vi "FPGA Top - Packet TX Only.vi"() -> ()   [LabVIEW 2020, in "My Network FPGA v1.lvlib"]
uses:
  My Network FPGA v1.lvlib
  <instrlib>/_niInstr/Network/Types/v1/MAC Address.ctl
  <instrlib>/_niInstr/Network/Types/v1/IPv4 Address.ctl
  <instrlib>/_niInstr/CLIP Adapters/v1/FPGA/AXI4-Lite/FXP32 Address - FXP32 Data/Public/CLIP Resources.ctl
  <vilib>/Platform/TimedLoop/XDataNode/timing_clust.ctl
  <vilib>/Platform/TimedLoop/XDataNode/nitl_modes.ctl
  <vilib>/Platform/TimedLoop/XDataNode/wakeup.ctl
  <instrlib>/_niInstr/Network/Ethernet/MAC/CLIP/v1/1GbE/Resources.ctl
  <instrlib>/_niInstr/FIFO Register Bus/v1/FPGA/niInstr FIFO Register Bus v1 FPGA.lvclass
  p:/lvdist/win32/export/20.0/20.0.0f2/dist/instr.lib/_niInstr/Instruction Framework/v1/FPGA/Interfaces/Instruction Producer/Instruction Producer.lvclass
  <instrlib>/_niInstr/CLIP Adapters/v1/FPGA/AXI4-Lite/Address Space Collection/niInstr AXI4-Lite Address Space Collection v1 FPGA.lvclass
  p:/lvdist/win32/export/20.0/20.0.0f2/dist/instr.lib/_niInstr/Instruction Framework/v1/FPGA/Interfaces/Address Space Collection/Address Space Collection.lvclass
  <vilib>/rvi/Emulation/niFpgaGetClockAttributes.vi
  <vilib>/rvi/Emulation/niFpgaSctlEmulationGetInTimedLoop.vi
  <vilib>/rvi/Emulation/niFpgaEmulationReportErrorSimple.vi
  <vilib>/rvi/Emulation/niFpgaCriticalErrorInLSC.vi
  <vilib>/rvi/DataTransferAndStorage/Container/Common/niFpgaContainerGetUniqueNameForEmu.vi
  <vilib>/rvi/DataTransferAndStorage/Container/Common/niFpgaContainerSetEmuInfo.vi
  <vilib>/rvi/eio/common/nirviEmuReportErrorAndStop.vi
  <vilib>/rvi/Emulation/niFpgaProcessEmulError.vi
  <vilib>/rvi/DataTransferAndStorage/Container/Common/niFpgaContainerExecOnDevCompGetState.vi
  <vilib>/rvi/Emulation/niFpgaEmulationIsFPGAContextNoSignature.vi
  <vilib>/rvi/errors/niFpgaSetErrorForExecOnDevCompSimple.vi
  <vilib>/rvi/FIFO/Fifo_Resource/nirvififoEmulationSetSize.vi
  <vilib>/rvi/FIFO/Fifo_Resource/nirviFifoEmulationQueueMgr.vi
  <instcachedir>/0/nirviFifoEmulationQueueMgr_E5CAEC123FF24DC58D834DCA3CDAA9B5.lvgen/nirviFifoEmulationQueueMgr_E5CAEC123FF24DC58D834DCA3CDAA9B5_022.vi
  <vilib>/rvi/FIFO/Fifo_Resource/nirvififoEmulationDetermineInputValidOut.vi
  <vilib>/rvi/FIFO/Fifo_Resource/nirvififoEmulationCreateLock.vi
  <vilib>/rvi/FIFO/Fifo_Resource/nirvififoEmulationObtainLock.vi
  <vilib>/rvi/FIFO/Fifo_Resource/nirvififoEmulationReleaseLock.vi
  <vilib>/rvi/occurrence/nirviWaitOnOccurrenceBase.vi
  <vilib>/rvi/errors/nirviReportUnexpectedCaseInternalError.vi
  <vilib>/rvi/errors/nirviReportUnexpectedCaseInternalError (U32).vi
  <vilib>/Utility/error.llb/Clear Errors.vi
  <vilib>/rvi/interface/RandomDataEmulation/niFpgaRandomDataHandleErrors.vi
  <vilib>/rvi/eio/common/nirviEmuTemplateMethod_errors.vi
  <vilib>/Platform/TimedLoop/XDataNode/XDataNode.xnode
  <vilib>/rvi/LocalResourceManager/LocalResourceManager.xnode
  <vilib>/rvi/DataTransferAndStorage/Container/XNode/niFpgaContainer.xnode
  <vilib>/rvi/FIFO/Fifo_Resource/niFpgaFifoEmulationRefIn.vi
  <vilib>/eio/EIONode/EIONode.xnode
  <instrlib>/_niInstr/Network/Ethernet/MAC/CLIP/v1/1GbE/niInstr Ethernet MAC - CLIP 1GbE v1.lvclass
  <instrlib>/_niInstr/Instruction Framework/v1/FPGA/Top Level Bus/Register Configuration/Register Configuration.lvclass
  <instrlib>/_niInstr/Network/Ethernet/MAC/Raw Stream/v1/niInstr Ethernet MAC Raw Stream v1.lvclass
  <vilib>/Platform/TimedLoop/XDataNode/XDNodeRunTimeDep.lvlib
  <instrlib>/_niInstr/Network/IPv4/UDP/FPGA/v1/niInstr IPv4 UDP FPGA v1.lvlib
  <instrlib>/_niInstr/CLIP Adapters/v1/FPGA/AXI4-Lite/FXP32 Address - FXP32 Data/niInstr AXI4-Lite - FXP32 Address - FXP32 Data v1 FPGA.lvclass
  <instrlib>/_niInstr/Network/Types/v1/niInstr Network Types v1.lvlib
panel:
  in  "fifo reg bus ctrl 0":u32
  out "fifo reg bus status 0":u32
  out "fifo reg bus data 0":u64
  in  "enable tx":bool=TRUE
  in  "max payload per frame":u16=1472
  in  "send packet":bool
  in  "udp payload length":u16=1024
  out "mgtrefclks_locked":bool
  out "mgtrefclks_valid":bool
  out "posc_complete":bool
  out "sPort0_Power_Good":bool
  out "sPort1_Power_Good":bool
  out "signal_detect_Port0":bool
  out "signal_detect_Port1":bool
  in  "UDP destination port":u16=35311
  in  "MAC destination address":T1=[255, 255, 255, 255, 255, 255] format="%.0x"
  in  "IPv4 destination address":T2=[255, 255, 255, 255]
  in  "UDP source port":u16
  in  "IPv4 source address":T2=[0, 0, 0, 0]
  in  "MAC source address":T1=[0, 128, 47, 0, 0, 1] format="%.0x"
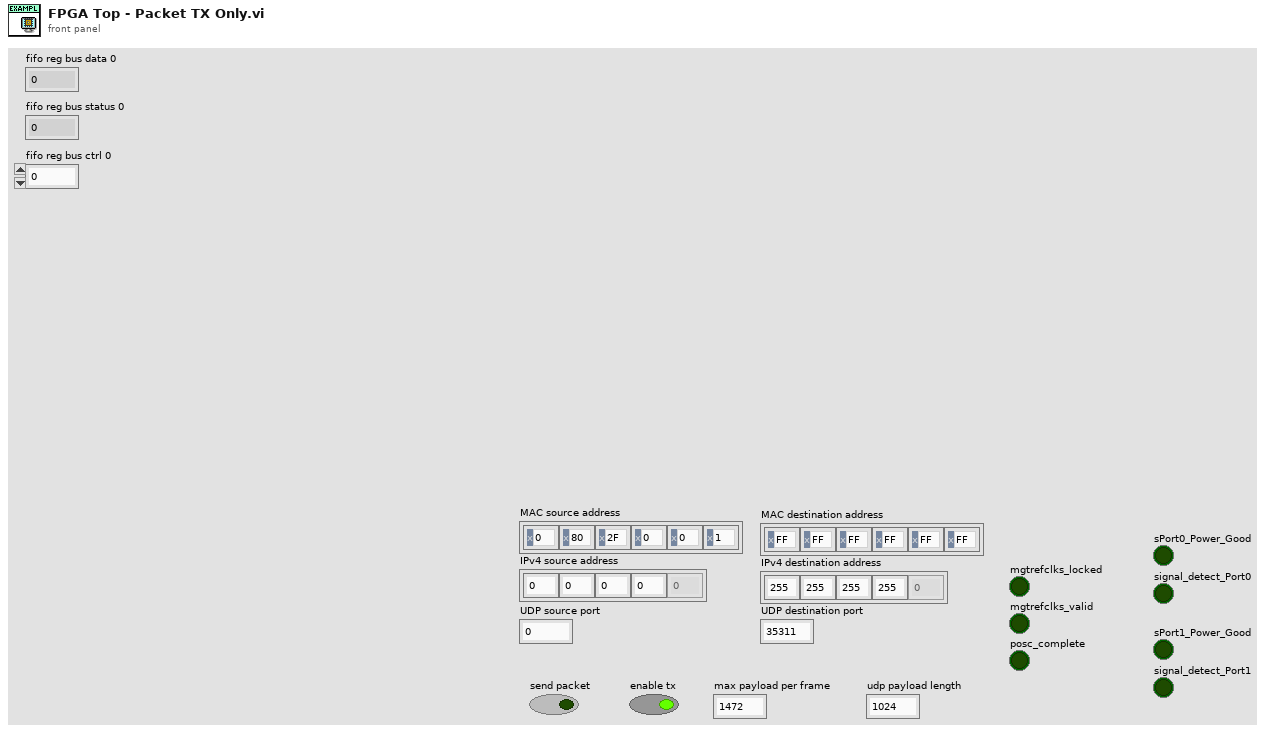
[diagram p1: front panel]
types:
  T1 = typedef "niInstr Network Types v1.lvlib/MAC Address.ctl" = u8[]
  T2 = typedef "niInstr Network Types v1.lvlib/IPv4 Address.ctl" = u8[]
  T3 = typedef "niInstr Ethernet MAC - CLIP 1GbE v1.lvclass/Resources.ctl" = cluster{"RX":cluster{"TData":refnum<k21>, "TValid":refnum<k21>, "TLast":refnum<k21>, "TUser":refnum<k21>}, "TX":cluster{"TData":refnum<k21>, "TValid":refnum<k21>, "TLast":refnum<k21>, "TUser":refnum<k21>, "TReady":refnum<k21>}, "Pause resources":cluster{"cPauseValuePort":refnum<k21>, "cPauseReqPort":refnum<k21>}, "MAC Clock":refnum<k21>}
  T4 = typedef "niInstr AXI4-Lite - FXP32 Address - FXP32 Data v1 FPGA.lvclass/CLIP Resources.ctl" = cluster{"s_axi_araddr":refnum<k21>, "s_axi_arvalid":refnum<k21>, "s_axi_arready":refnum<k21>, "s_axi_rdata":refnum<k21>, "s_axi_rresp":refnum<k21>, "s_axi_rvalid":refnum<k21>, "s_axi_rready":refnum<k21>, "s_axi_awaddr":refnum<k21>, "s_axi_awvalid":refnum<k21>, "s_axi_awready":refnum<k21>, "s_axi_wdata":refnum<k21>, "s_axi_wstrb":refnum<k21>, "s_axi_wvalid":refnum<k21>, "s_axi_wready":refnum<k21>, "s_axi_bresp":refnum<k21>, "s_axi_bvalid":refnum<k21>, "s_axi_bready":refnum<k21>}
  T5 = typedef "XDNodeRunTimeDep.lvlib/timing_clust.ctl" = cluster{"Expected End [f-1]":u64, "Actual End [f-1]":u64, "Finished Late? [f-1]":bool, "Expected End [i-1]":u64, "Actual End [i-1]":u64, "Finished Late? [i-1]":bool, "Expected Start [i]":u64, "Actual Start [i]":u64, "Expected Start [f]":u64, "Actual Start [f]":u64, "Source Name":string, "Structure Name":string, "Period":i64, "Deadline":i64, "Offset":i64, "Start":i64, "Priority":i32, "Timeout":i32, "Mode":T6, "Wakeup Reason":T7, "Error":errorcluster, "Source Type":string, "Secondary Source Type":string, "Global End Time":u64, "Global Start Time":u64, "Frame Duration":u64, "Iteration Duration":u64, "Assigned CPU":i32, "I/O Scan Engine Mode":u32}
  T6 = typedef "XDNodeRunTimeDep.lvlib/nitl_modes.ctl" = enum32{"No Change", "Process missed periods, maintain original phase", "Discard missed periods, maintain original phase", "Process missed periods, ignore original phase", "Discard missed periods, ignore original phase"}
  T7 = typedef "XDNodeRunTimeDep.lvlib/wakeup.ctl" = enum32{"Normal", "Aborted", "Asynchronous wakeup", "Timing source error", "Timed loop error", "Timeout"}
  T8 = cluster{"ready for input (payload data)":bool, "ready for input (start packet)":bool}
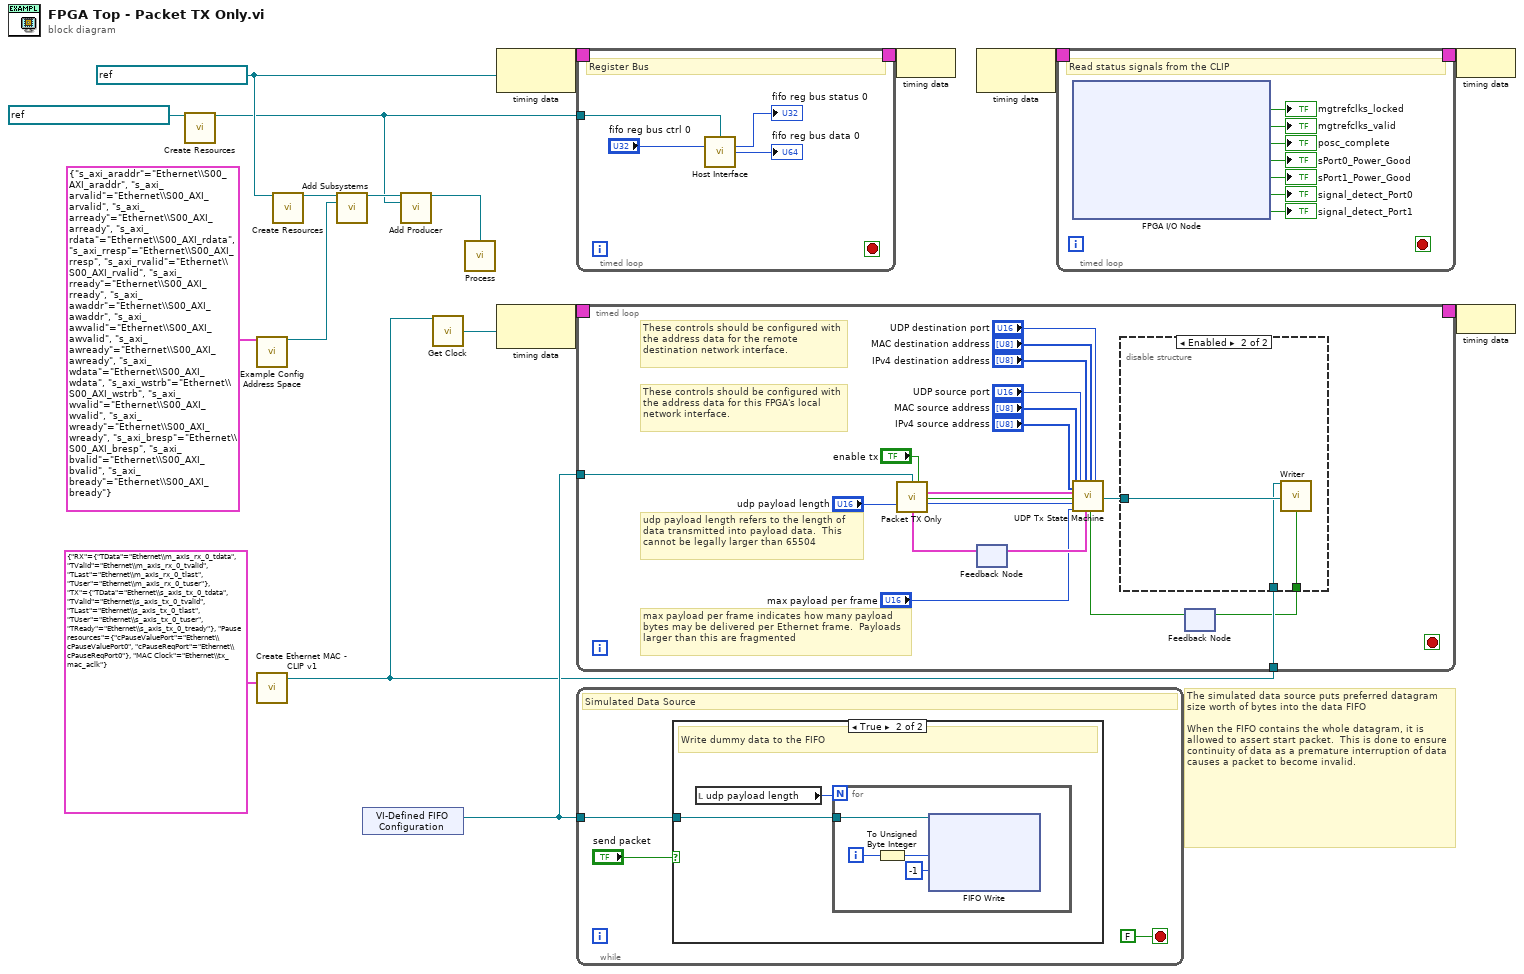
[diagram p0: block diagram]
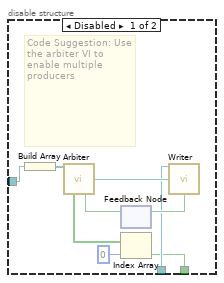
[diagram p3: hidden frame]
diagram:
  w8 = refnum<k21> "40 MHz Onboard Clock" ("Source Name")
  # "The simulated data source puts preferred datagram size worth of bytes into the data FIFO\n\nWhen the FIFO contains the whole datagram, it is allowed to assert start packet.  This is done to ensure continuity of data as a premature interruption of data causes a packet to become invalid."
  n1 = call <instrlib>:"Create Resources.vi"("instruction fifo"=refnum<k21> "reg.host instruction fifo 0" ("FIFO")) -> ("fifo register bus"=w3:refnum<class "niInstr FIFO Register Bus v1 FPGA.lvclass">)  [unwired: 14 in]
  n2 = call "Example Config Address Space.vi"("clip resources in"=T4 {"s_axi_araddr"="Ethernet\\S00_AXI_araddr", "s_axi_arvalid"="Ethernet\\S00_AXI_arvalid", "s_axi_arready"="Ethernet\\S00_AXI_arready", "s_axi_rdata"="Ethernet\\S00_AXI_rdata", "s_axi_rresp"="Ethernet\\S00_AXI_rresp", "s_axi_rvalid"="Ethernet\\S00_AXI_rvalid", "s_axi_rready"="Ethernet\\S00_AXI_rready", "s_axi_awaddr"="Ethernet\\S00_AXI_awaddr", "s_axi_awvalid"="Ethernet\\S00_AXI_awvalid", "s_axi_awready"="Ethernet\\S00_AXI_awready", "s_axi_wdata"="Ethernet\\S00_AXI_wdata", "s_axi_wstrb"="Ethernet\\S00_AXI_wstrb", "s_axi_wvalid"="Ethernet\\S00_AXI_wvalid", "s_axi_wready"="Ethernet\\S00_AXI_wready", "s_axi_bresp"="Ethernet\\S00_AXI_bresp", "s_axi_bvalid"="Ethernet\\S00_AXI_bvalid", "s_axi_bready"="Ethernet\\S00_AXI_bready"}) -> ("MAC Configuration Address Space"=w4:refnum<class "niInstr AXI4-Lite Address Space Collection v1 FPGA.lvclass">)  [unwired: 14 in]
  n3 = call <instrlib>:"Create Ethernet MAC - CLIP v1.vi"("Ethernet AXI4-S Resources"=T3 {"RX"={"TData"="Ethernet\\m_axis_rx_0_tdata", "TValid"="Ethernet\\m_axis_rx_0_tvalid", "TLast"="Ethernet\\m_axis_rx_0_tlast", "TUser"="Ethernet\\m_axis_rx_0_tuser"}, "TX"={"TData"="Ethernet\\s_axis_tx_0_tdata", "TValid"="Ethernet\\s_axis_tx_0_tvalid", "TLast"="Ethernet\\s_axis_tx_0_tlast", "TUser"="Ethernet\\s_axis_tx_0_tuser", "TReady"="Ethernet\\s_axis_tx_0_tready"}, "Pause resources"={"cPauseValuePort"="Ethernet\\cPauseValuePort0", "cPauseReqPort"="Ethernet\\cPauseReqPort0"}, "MAC Clock"="Ethernet\\tx_mac_aclk"}) -> ("niInstr Ethernet MAC - CLIP 1GbE v1.lvclass out"=w1:refnum<class "niInstr Ethernet MAC - CLIP 1GbE v1.lvclass">)  [unwired: 14 in]
  n4 = call <instrlib>:"Create Resources.vi"("register clock"=w8) -> ("register configuration"=w5:refnum<class "Register Configuration.lvclass">)  [unwired: 14 in]
  n5 = call-dynamic "Add Subsystems.vi"("register configuration in"=w5, "subsystems"=w4) -> ("register configuration out"=w6:refnum<class "Register Configuration.lvclass">)  [unwired: 13 in]
  n6 = xnode "VI-Defined FIFO Configuration"() -> ("FIFO Out"=w16:refnum<k21>)
  n7 = call-dynamic "Add Producer.vi"("register configuration in"=w6, "instruction producer"=w3) -> ("register configuration out"=w7:refnum<class "Register Configuration.lvclass">)  [unwired: 13 in]
  n8 = call-dynamic "Get Clock.vi"("niInstr Ethernet MAC - CLIP v1.lvclass"=w1) -> ("MAC Clock"=w13:refnum<k21>)  [unwired: 14 in]
  n9 = call-dynamic "Process.vi"("register configuration"=w7) -> ()  [unwired: 15 in]
  n10 = node-c288(w8) -> (w12:T5)
  n11 = node-c288(w13) -> (w18:T5)
  n12 = timed-loop {
    timing: w12 -> [_]
    timing-out: [_] -> w11
    tunnel: w3 -> [w22]
    stop <- _ stop-if-true
    # "Register Bus"
    n13 = call <instrlib>:"Host Interface.vi"("fifo register bus"=w22, "fifo reg bus ctrl 0"="fifo reg bus ctrl 0") -> ("fifo reg bus status 0"=→"fifo reg bus status 0":u32, "fifo reg bus data 0"=→"fifo reg bus data 0":u64)  [unwired: 12 in]
  }
  n14 = timed-loop {
    timing: w18 -> [_]
    timing-out: [_] -> w17
    tunnel: w1 -> [w43]
    tunnel: w16 -> [w30]
    stop <- _ stop-if-true
    # "udp payload length refers to the length of data transmitted into payload data.  This cannot be legally larger than 65504"
    # "max payload per frame indicates how many payload bytes may be delivered per Ethernet frame.  Payloads larger than this are fragmented"
    # "These controls should be configured with the address data for this FPGA's local network interface."
    # "These controls should be configured with the address data for the remote destination network interface."
    n15 = feedback #1() -> (w29:T8)  [unwired: 1 in]
    n16 = call "Packet TX Only.vi"("payload fifo"=w30, "enable tx"="enable tx", "udp payload length"="udp payload length", "ready for input"=w29) -> ("payload data"=w26:cluster{"Element":u8[], "Output Valid":bool}, "start packet"=w27:bool, "payload length"=w28:u16)  [unwired: 9 in]
    n17 = feedback #2() -> (w39:bool)  [unwired: 1 in]
    n18 = call <instrlib>:"UDP Tx State Machine.vi"("MAC source address"="MAC source address", "IPv4 source address"="IPv4 source address", "payload data"=w26, "start packet"=w27, "payload length"=w28, "max payload per frame"="max payload per frame", "UDP source port"="UDP source port", "IPv4 destination address"="IPv4 destination address", "MAC destination address"="MAC destination address", "ready for output"=w39, "UDP destination port"="UDP destination port") -> ("ready for input"=w40:T8, "niInstr Ethernet MAC Raw Stream v1 out"=w42:refnum<class "niInstr Ethernet MAC Raw Stream v1.lvclass">)  [unwired: 7 in]
    n19 = feedback-in #1(w40) -> ()
    n20 = disable-structure shown="Enabled" {
      disable-tunnel: w43 -> [w48 w53]
      disable-tunnel: w42 -> [w46 w54]
      disable-tunnel: [w45 w55] -> w41
      frame Disabled {
        # "Code Suggestion: Use the arbiter VI to enable multiple producers"
        n21 = Build Array(w46) -> (w47:refnum<class "niInstr Ethernet MAC Raw Stream v1.lvclass">[])
        n22 = feedback #3() -> (w50:bool)  [unwired: 1 in]
        n23 = call <instrlib>:"Arbiter.vi"("inbound packet streams"=w47, "ready for output"=w50) -> ("element"=w52:refnum<class "niInstr Ethernet MAC Raw Stream v1.lvclass">, "ready for input"=w51:bool[])  [unwired: 12 in]
        n24 = Index Array(array=w51, index=0) -> (element=w45:bool)
        n25 = call-dynamic "Writer.vi"("niInstr Ethernet MAC v1.lvclass"=w48, "niInstr Ethernet MAC Raw Stream v1.lvclass"=w52) -> ("ready for input?"=w49:bool)  [unwired: 12 in, 1 out]
        n26 = feedback-in #3(w49) -> ()
      }
      frame Enabled {
        n27 = call-dynamic "Writer.vi"("niInstr Ethernet MAC v1.lvclass"=w53, "niInstr Ethernet MAC Raw Stream v1.lvclass"=w54) -> ("ready for input?"=w55:bool)  [unwired: 12 in, 1 out]
      }
    }
    n28 = feedback-in #2(w41) -> ()
  }
  n29 = while {
    tunnel: w16 -> [w59]
    stop <- FALSE stop-if-true
    # "Simulated Data Source"
    n30 = case shown="True" "send packet" {
      tunnel: w59 -> [_ w61]
      frame False {
      }
      frame True {
        # "Write dummy data to the FIFO"
        n31 = local read "udp payload length"() -> (w62:u16)
        n32 = for {
          N: w62 -> [_]
          tunnel: w61 -> [w66]
          i -> [w64]
          n33 = To Unsigned Byte Integer(number=w64) -> (unsigned 8bit integer=w63:u8)
          n34 = xnode ("FIFO Write")("Element"=w63, "Timeout"=-1, "FIFO In"=w66) -> ()  [unwired: 2 out]
        }
      }
    }
  }
  n35 = node-c288(w11) -> ()
  n36 = node-c288() -> (w15:T5)  [unwired: 1 in]
  n37 = timed-loop {
    timing: w15 -> [_]
    timing-out: [_] -> w14
    stop <- _ stop-if-true
    # "Read status signals from the CLIP"
    n38 = xnode "FPGA I/O Node"() -> ("Ethernet\\MgtRefClks_Locked"=→"mgtrefclks_locked":bool, "Ethernet\\MgtRefClks_Valid"=→"mgtrefclks_valid":bool, "Ethernet\\POSC_Complete"=→"posc_complete":bool, "Ethernet\\sPort0_Power_Good"=→"sPort0_Power_Good":bool, "Ethernet\\sPort1_Power_Good"=→"sPort1_Power_Good":bool, "Ethernet\\signal_detect_Port0"=→"signal_detect_Port0":bool, "Ethernet\\signal_detect_Port1"=→"signal_detect_Port1":bool)  [unwired: 7 in, 7 out]
  }
  n39 = node-c288(w14) -> ()
  n40 = node-c288(w17) -> ()
